vi "DVR Unflatten.vi"(8 "error in (no error)":errorcluster, 10 "DVRs In":refnum<data-value>[](array[refnum]), 11 "Flatten Data in":u8[](array[numeric])) -> (0 "error out":errorcluster, 2 "DVRs Out":refnum<data-value>[](array[refnum]), 3 "Flatten Data out":u8[](array[numeric]), 5 "Header out":T1)   [LabVIEW 2021]
uses:
  typedef/FIFO Header.ctl
  typedef/Datatype Waveform.ctl
  typedef/Errors.ctl
  <vilib>/CIF Foundation/CIF Utilities/DataTypes/Unflatten I64.vi
  <vilib>/CIF Foundation/CIF Utilities/Errors/Append Error Location.vi
  ChannelCommon.lvlib
  <vilib>/CIF Foundation/CIF Utilities/DataTypes/DataTypes_CIF_U.lvlib
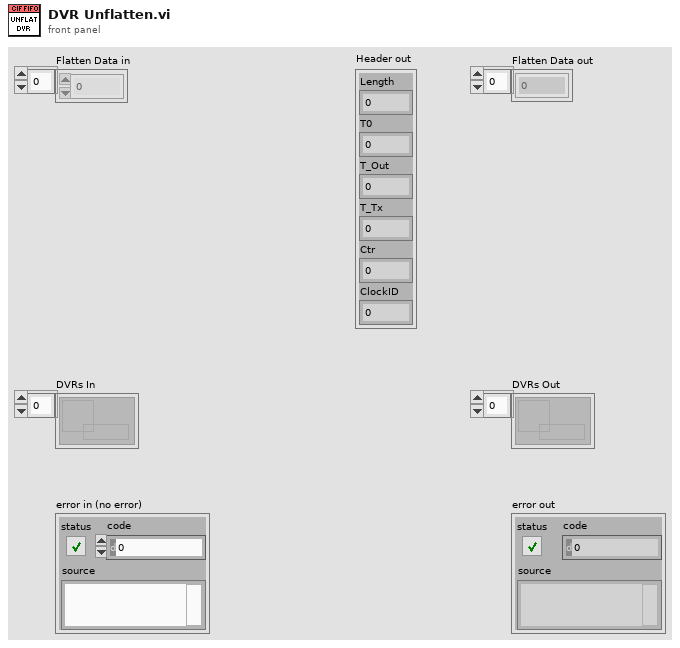
[diagram p1: front panel]
types:
  T1 = typedef "ChannelCommon.lvlib/FIFO Header.ctl" = cluster{"Length":u64, "T0":i64, "T_Out":i64, "T_Tx":i64, "Ctr":u64, "ClockID":u8}
  T2 = typedef "ChannelCommon.lvlib/Errors.ctl" = enum16{"gRPC Server Not Found", "Duplicate Channel", "Missing Channel", "Incorrect Type", "Flatten Error", "Unflatten Data", "Channel Length", "Plugin Connection", "gRPC Server Connection", "FIFO Unflatten"}
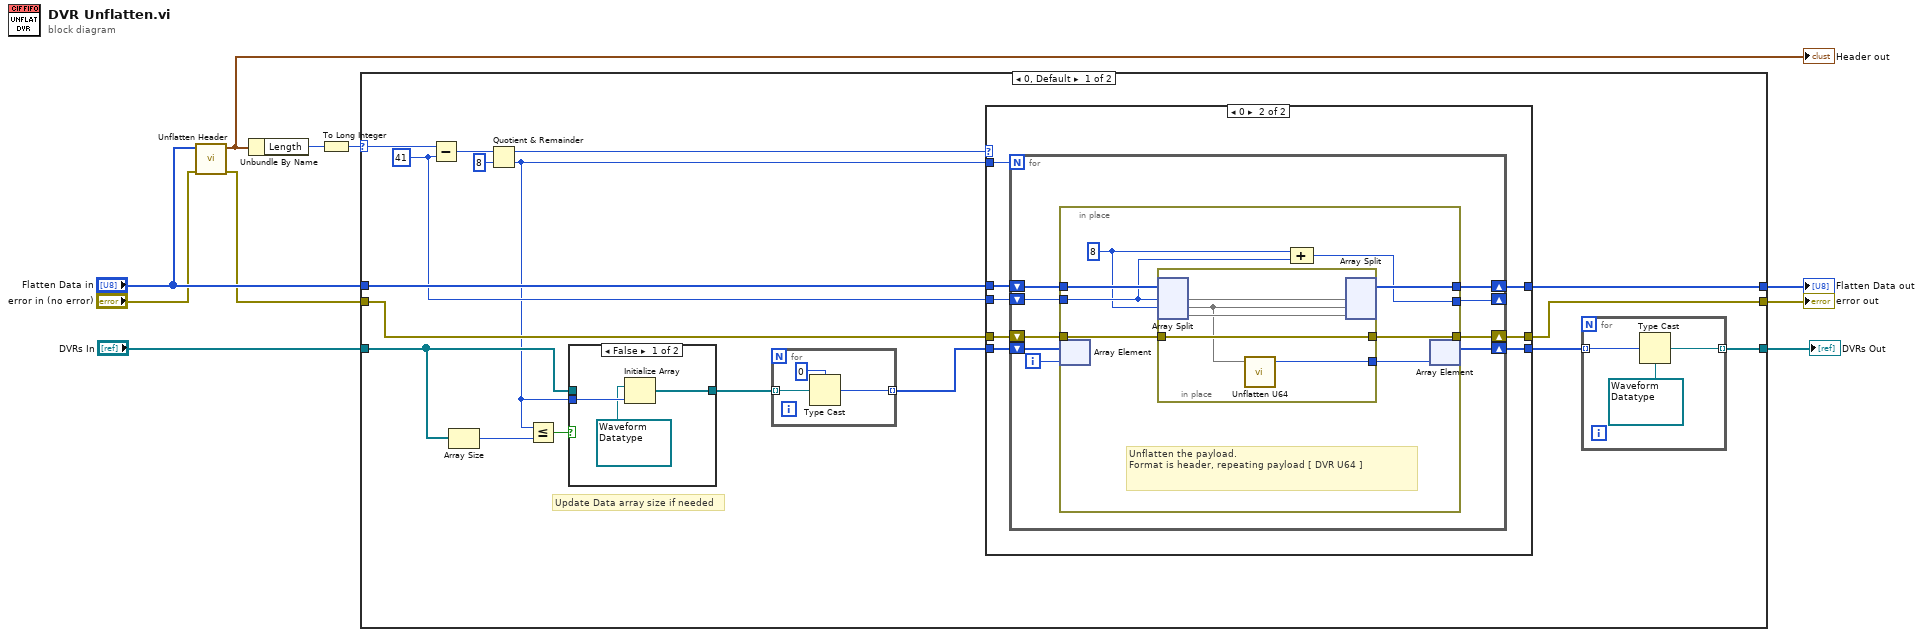
[diagram p0: block diagram]
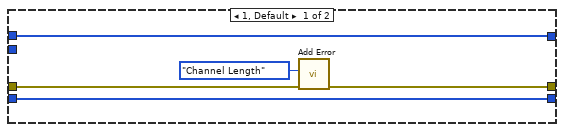
[diagram p2: hidden frame]
diagram:
  n1 = call "Unflatten Header.vi"("error in (no error)"="error in (no error)", "Flattened Data in"="Flatten Data in") -> ("error out"=w1:errorcluster, "Header out"=w7:T1)  [unwired: 7 in, 1 out]
  "Header out" <- w7
  n2 = Unbundle By Name(w7) -> ("Length"=w8:u64)
  n3 = To Long Integer(number=w8) -> (32bit integer=w6:i32)
  n4 = case shown="0, Default" w6 {
    selector: w6 -> [w23 _]
    tunnel: [w11 w73] -> w4
    tunnel: "DVRs In" -> [w17 w73]
    tunnel: [w27 w74] -> w10
    tunnel: [w26 w75] -> w9
    tunnel: "Flatten Data in" -> [w25 w75]
    tunnel: w1 -> [w24 w74]
    frame 0, Default {
      w22 = 41
      # "Update Data array size if needed"
      n5 = Subtract(x=w23, y=w22) -> (x-y=w21:i32)
      n6 = Array Size(array=w17) -> (size(s)=w19:i32)
      n7 = Quotient & Remainder(x=w21, y=8) -> (x-y*floor(x/y)=w15:i32, floor(x/y)=w16:i32)
      n8 = Less Or Equal?(x=w16, y=w19) -> (x <= y?=w18:bool)
      n9 = case shown="False" w18 {
        tunnel: w17 -> [_ w72]
        tunnel: [w71 w72] -> w14
        tunnel: w16 -> [w70 _]
        frame False {
          n10 = Initialize Array(refnum<data-value> refnum ("element"), w70) -> (w71:refnum<data-value>[])
        }
        frame True {
        }
      }
      n11 = for {
        tunnel: w14 -> [w33] mode=indexing
        tunnel: [w31] -> w13 mode=indexing
        n12 = Type Cast(type=u64 0, x=w33) -> (*(type *) &x=w31:u64)
      }
      n13 = case shown="0" w15 {
        tunnel: [w36 w46] -> w12
        tunnel: [w35 w45] -> w27
        tunnel: [w38 w44] -> w26
        tunnel: w25 -> [w38 w43]
        tunnel: w24 -> [w37 w42]
        tunnel: w22 -> [_ w41]
        tunnel: w13 -> [w36 w40]
        tunnel: w16 -> [_ w39]
        frame 1, Default {
          n14 = call "Add Error.vi"("error in (no error)"=w37, "Error"=Errors."Channel Length") -> ("error out"=w35:errorcluster)  [unwired: 9 in]
        }
        frame 0 {
          n15 = for {
            N: w39 -> [_]
            shift-right: [w47] -> w45
            shift-left: w42 -> [w52]
            shift-right: [w55] -> w44
            shift-left: w43 -> [w54]
            shift-right: [w51] -> _
            shift-left: w41 -> [w53]
            shift-right: [w48] -> w46
            shift-left: w40 -> [w49]
            i -> [w50]
            n16 = in-place {
              in-place-border: [w63] -> w55
              in-place-border: w54 -> [w62]
              in-place-border: w53 -> [w61]
              in-place-border: w52 -> [w60]
              in-place-border: [w59] -> w51
              in-place-border: [w56] -> w47
              w58 = 8 ("y")
              # "Unflatten the payload.\nFormat is header, repeating payload [ DVR U64 ]"
              n17 = in-place-array #1(w49, w50) -> ()  [unwired: 1 out]
              n18 = in-place {
                in-place-border: [w66] -> w57
                in-place-border: w60 -> [w65]
                in-place-border: [w65] -> w56
                n19 = in-place-split #2(w62, w61, w58) -> (w68:u8[], w64:u8[], w67:u8[])
                n20 = call <vilib>:"Unflatten U64.vi"("Flat Data"=w64) -> ("U64"=w66:u64)  [unwired: 4 in]
                n21 = in-place-split #2(w68, w64, w67) -> (w63:u8[])  [unwired: 2 out]
              }
              n22 = Compound Arithmetic op=ADD(w58, w61) -> (w59:i32)
              n23 = in-place-array #1(w57) -> (w48:u64[])  [unwired: 1 out]
            }
          }
        }
      }
      n24 = for {
        tunnel: w12 -> [w30] mode=indexing
        tunnel: [w29] -> w11 mode=indexing
        n25 = Type Cast(type=refnum<data-value> refnum ("element"), x=w30) -> (*(type *) &x=w29:refnum<data-value>)
      }
    }
    frame 40 {
      # "Header only"
    }
  }
  "error out" <- w10
  "Flatten Data out" <- w9
  "DVRs Out" <- w4
